vi "_Open Preference File.vi"(4 "error In":errorcluster, 6 "Initialize":bool, 7 "Server":bool) -> (0 "error":errorcluster, 2 "ipf path":path, 3 "refnum":T1)   [LabVIEW 2015]
uses:
  <vilib>/Utility/config.llb/Config Data RefNum.ctl
  <vilib>/Utility/config.llb/NI_LVConfig.lvlib
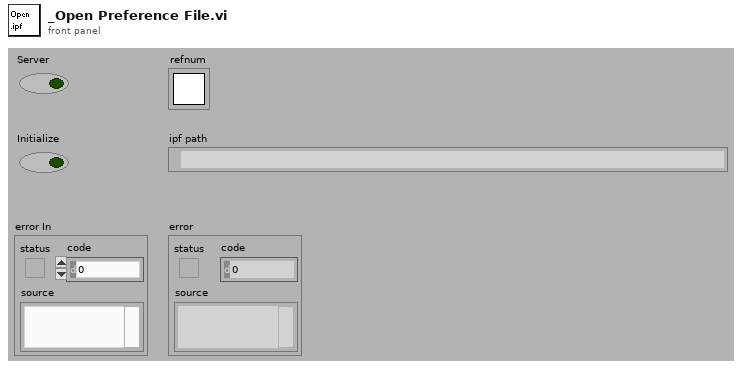
[diagram p1: front panel]
types:
  T1 = typedef "NI_LVConfig.lvlib/Config Data RefNum.ctl" = refnum<k1>
  T2 = enum32{"existing file", "new file", "new or existing file", "existing dir", "new dir", "new or existing dir", "existing file (use LLBs)", "new file (use LLBs)", "new or existing file (use LLBs)", "new or existing file or directory (use LLBs)"}
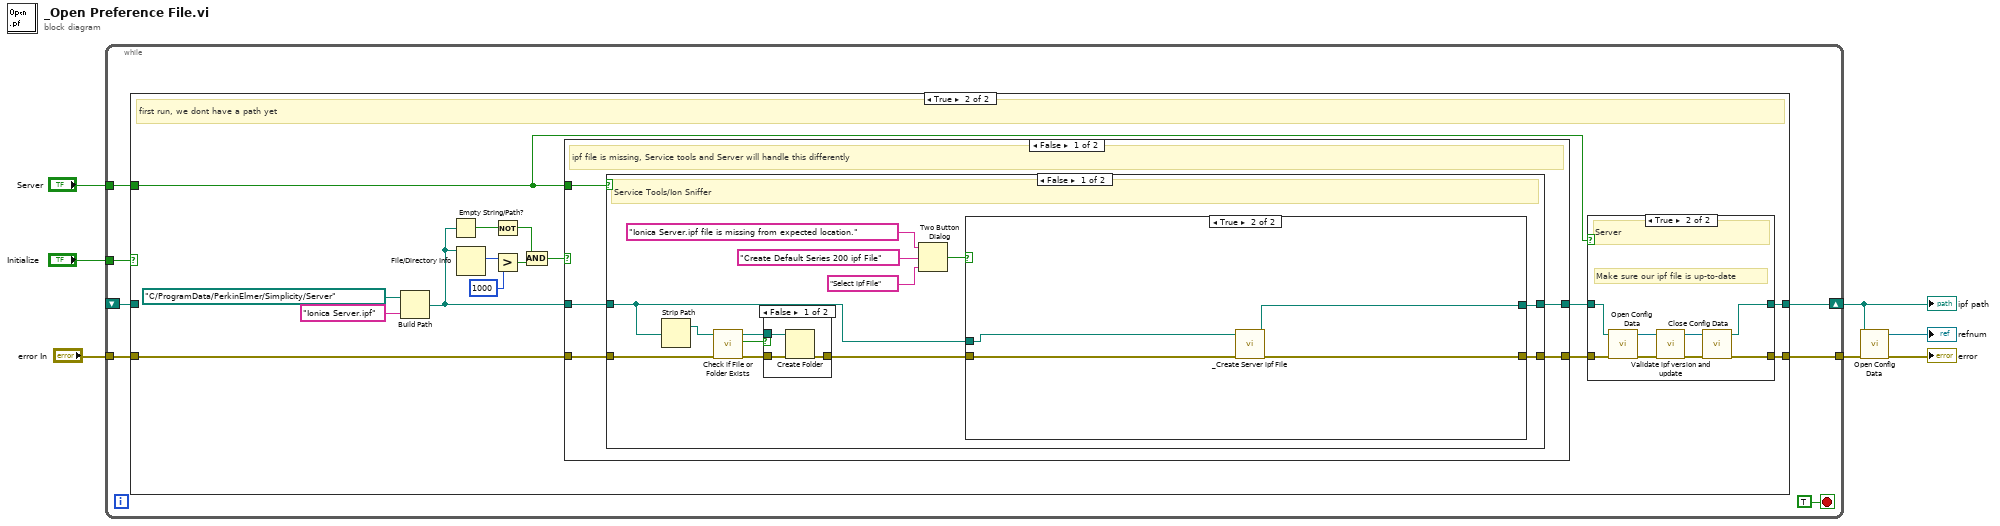
[diagram p0: block diagram]
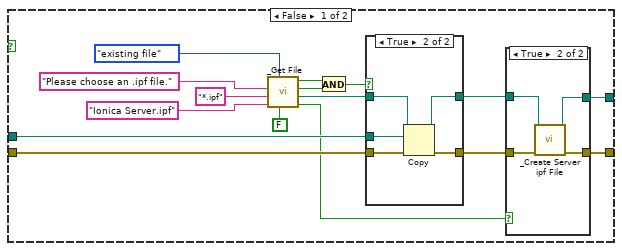
[diagram p4: hidden frame]
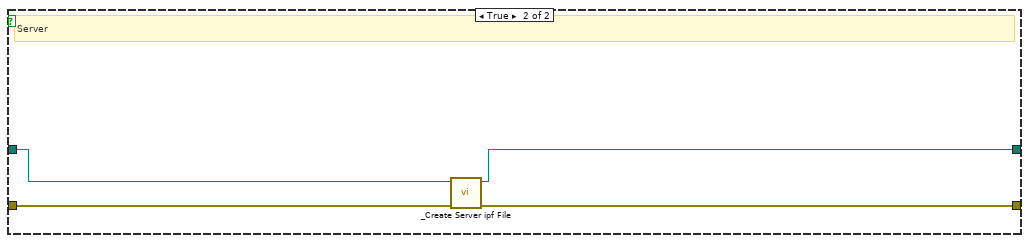
[diagram p8: hidden frame]
diagram:
  n1 = while {
    tunnel: "Server" -> [w13]
    shift-right: [w14] -> w7
    shift-left: _ -> [w10]
    tunnel: "Initialize" -> [w12]
    tunnel: "error In" -> [w9]
    tunnel: [w8] -> w1
    stop <- TRUE stop-if-true
    n2 = case shown="True" w12 {
      tunnel: [w16 w19] -> w14
      tunnel: w13 -> [_ w17]
      tunnel: w10 -> [w16 _]
      tunnel: w9 -> [w15 w22]
      tunnel: [w15 w20] -> w8
      frame False {
        # "we already have a file path, use it"
      }
      frame True {
        # "first run, we dont have a path yet"
        n3 = Build Path(base path=path "C:/ProgramData/PerkinElmer/Simplicity/Server" ("appended path"), name or relative path="Ionica Server.ipf") -> (appended path=w29:path)
        n4 = Empty String/Path?(string/path=w29) -> (empty?=w25:bool)
        n5 = File/Directory Info(path=w29) -> (size=w27:i64)  [unwired: 1 in, 6 out]
        n6 = Not(x=w25) -> (.not. x?=w26:bool)
        n7 = Greater?(x=w27, y=i64 1000) -> (0:w24:bool)
        n8 = And(x=w26, y=w24) -> (x .and. y?=w23:bool)
        n9 = case shown="False" w23 {
          tunnel: [w46 w102] -> w18
          tunnel: w29 -> [w45 w102]
          tunnel: w17 -> [w44 _]
          tunnel: w22 -> [w43 w101]
          tunnel: [w42 w101] -> w21
          frame False {
            # "ipf file is missing, Service tools and Server will handle this differently"
            n10 = case shown="False" w44 {
              tunnel: [w51 w97] -> w46
              tunnel: w45 -> [w54 w100]
              tunnel: w43 -> [w59 w99]
              tunnel: [w52 w98] -> w42
              frame False {
                # "Service Tools/Ion Sniffer"
                n11 = Strip Path(path=w54) -> (stripped path=w53:path)  [unwired: 1 out]
                n12 = call <vilib>:"Check if File or Folder Exists.vi"("error in (no error)"=w59, "path"=w53) -> ("error out"=w58:errorcluster, "file or folder exists?"=w55:bool, "dup path"=w56:path)  [unwired: 7 in]
                n13 = case shown="False" w55 {
                  tunnel: w58 -> [w95 w96]
                  tunnel: [w94 w96] -> w57
                  tunnel: w56 -> [w93 _]
                  frame False {
                    n14 = Create Folder(path (use dialog)=w93, error in=w95) -> (error out=w94:errorcluster)  [unwired: 1 in, 2 out]
                  }
                  frame True {
                  }
                }
                n15 = Two Button Dialog(message="Ionica Server.ipf file is missing from expected location.", 1:"Select ipf File" ("T button name (\"OK\")"), 2:"Create Default Series 200 ipf File" ("T button name (\"OK\")")) -> (T button?=w47:bool)
                n16 = case shown="True" w47 {
                  tunnel: w57 -> [w66 w92]
                  tunnel: w54 -> [w65 w91]
                  tunnel: [w63 w89] -> w52
                  tunnel: [w61 w90] -> w51
                  frame False {
                    n17 = call "_Get File.vi"("For Write (T)"=FALSE, "select mode (new or existing)"=T2."existing file", "default name"="Ionica Server.ipf", "extension (isd)"="*.ipf", "prompt"="Please choose an .ipf file.") -> ("cancelled"=w60:bool, "Seleted File"=w67:path, "Exists"=w69:bool, "Succeeded"=w70:bool)  [unwired: 1 in]
                    n18 = And(x=w70, y=w69) -> (x .and. y?=w68:bool)
                    n19 = case shown="True" w68 {
                      tunnel: w67 -> [_ w88]
                      tunnel: w65 -> [w83 w87]
                      tunnel: [w83 w86] -> w62
                      tunnel: w66 -> [w82 w85]
                      tunnel: [w82 w84] -> w64
                      frame False {
                      }
                      frame True {
                        n20 = Copy(8:w85, 10:w87, 11:w88) -> (0:w84:errorcluster, 3:w86:path)  [unwired: 2 in, 1 out]
                      }
                    }
                    n21 = case shown="True" w60 {
                      tunnel: w64 -> [w77 w81]
                      tunnel: [w77 w80] -> w63
                      tunnel: w62 -> [w76 w79]
                      tunnel: [w76 w78] -> w61
                      frame False {
                      }
                      frame True {
                        n22 = call "_Create Server ipf File.vi"("error in"=w81, "Default ipf file path"=w79) -> ("error out"=w80:errorcluster, "ipf file path"=w78:path)  [unwired: 8 in]
                      }
                    }
                  }
                  frame True {
                    n23 = call "_Create Server ipf File.vi"("error in"=w92, "Default ipf file path"=w91) -> ("error out"=w89:errorcluster, "ipf file path"=w90:path)  [unwired: 8 in]
                  }
                }
              }
              frame True {
                # "Server"
                n24 = call "_Create Server ipf File.vi"("error in"=w99, "Default ipf file path"=w100) -> ("error out"=w98:errorcluster, "ipf file path"=w97:path)  [unwired: 8 in]
              }
            }
          }
          frame True {
            # ".ipf File found use it"
          }
        }
        n25 = case shown="True" w17 {
          tunnel: w21 -> [w32 w37]
          tunnel: [w32 w36] -> w20
          tunnel: [w33 w35] -> w19
          tunnel: w18 -> [w33 w34]
          frame False {
            # "Service Tool"
          }
          frame True {
            # "Make sure our ipf file is up-to-date"
            # "Server"
            n26 = call <vilib>:"Open Config Data.vi"("error in (no error)"=w37, "configuration file path"=w34) -> ("error out"=w40:errorcluster, "refnum"=w41:T1)  [unwired: 7 in, 1 out]
            n27 = call "Validate ipf version and update.vi"("error In"=w40, "refnum In"=w41) -> ("error Out"=w38:errorcluster, "refnum Out"=w39:T1)  [unwired: 8 in]
            n28 = call <vilib>:"Close Config Data.vi"("error in (no error)"=w38, "refnum"=w39) -> ("error out"=w36:errorcluster, "file path"=w35:path)  [unwired: 8 in]
          }
        }
      }
    }
  }
  "ipf path" <- w7
  n29 = call <vilib>:"Open Config Data.vi"("error in (no error)"=w1, "configuration file path"=w7) -> ("error out"=→"error":errorcluster, "refnum"=→"refnum":T1)  [unwired: 7 in, 1 out]
